vi "Initialize Module.vi"(8 "error in (no error)":errorcluster, 9 "Initialize on Error?":bool, 10 "configuration in":refnum<class "TBM module configuration.lvclass">, 11 "TBM module execution interface in":refnum<class "TBM module execution interface.lvclass">) -> (0 "error out":errorcluster, 1 "data allocations":T2, 2 "execution settings":T1, 3 "TBM module execution interface out":refnum<class "TBM module execution interface.lvclass">)   [LabVIEW 2013, in "Standard Engine Runtime.lvclass"]
uses:
  Standard Engine Runtime.lvclass
  <vilib>/NI/Tag Bus Module Framework/module configuration/TBM module configuration.lvclass
  <vilib>/NI/Tag Bus Module Framework/runtime/TBM module execution interface.lvclass
  <vilib>/NI/Tag Bus Module Framework/channel/data tables.ctl
  <vilib>/NI/Tag Bus/dictionary/data dictionary.lvclass
  <vilib>/NI/Tag Bus/dictionary table pair.ctl
  <vilib>/NI/Tag Bus/table/data table.ctl
  <vilib>/NI/Tag Bus Module Framework/runtime/execution settings.ctl
  <vilib>/NI/Tag Bus/table/data table.lvlib
  <vilib>/NI/Tag Bus/tag bus.lvlib
  <vilib>/NI/Tag Bus Module Framework/channel/TBM channel.lvclass
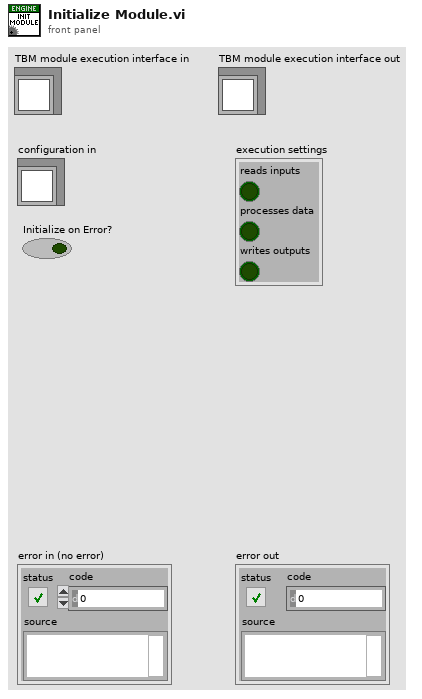
[diagram p1: front panel]
types:
  T1 = typedef "TBM module execution interface.lvclass/execution settings.ctl" = cluster{"reads inputs":bool, "processes data":bool, "writes outputs":bool}
  T2 = typedef "TBM channel.lvclass/data tables.ctl" = cluster{"input data":T3, "processing parameter":T3, "processing result":T3, "output data":T3}
  T3 = typedef "tag bus.lvlib/dictionary table pair.ctl" = cluster{"data dictionary":refnum<class "data dictionary.lvclass">, "data table":T4}
  T4 = typedef "tag bus.lvlib/data table.lvlib/data table.ctl" = cluster{"Double":dbl[], "Single":sgl[], "I64":i64[], "I32":i32[], "I16":i16[], "I8":i8[], "U64":u64[], "U32":u32[], "U16":u16[], "U8":u8[], "Boolean":bool[], "String":string[], "Array of Double":cluster{"DBL Array":dbl[]}[], "Array of Single":cluster{"SGL Array":sgl[]}[], "Array of I64":cluster{"I64 Array":i64[]}[], "Array of I32":cluster{"I32 Array":i32[]}[], "Array of I16":cluster{"I16 Array":i16[]}[], "Array of I8":cluster{"I8 Array":i8[]}[], "Array of U64":cluster{"U64 Array":u64[]}[], "Array of U32":cluster{"U32 Array":u32[]}[], "Array of U16":cluster{"U16 Array":u16[]}[], "Array of U8":cluster{"U8 Array":u8[]}[], "Array of Boolean":cluster{"Boolean Array":bool[]}[], "Array of String":cluster{"String Array":string[]}[]}
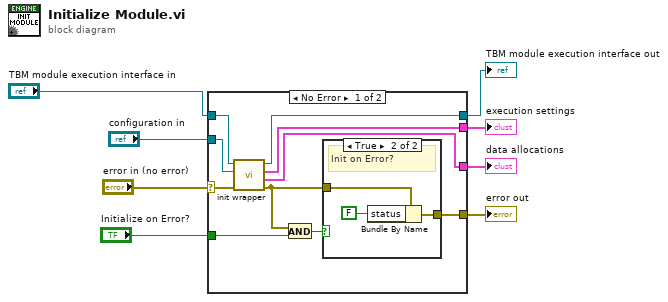
[diagram p0: block diagram]
diagram:
  n1 = case shown="No Error" "error in (no error)" {
    selector: "error in (no error)" -> [w9 w24]
    tunnel: [w18 w24] -> w8
    tunnel: "Initialize on Error?" -> [w15 _]
    tunnel: "configuration in" -> [w14 _]
    tunnel: [w13 w23] -> w5
    tunnel: [w12 _] -> w4
    tunnel: [w11 _] -> w3
    tunnel: "TBM module execution interface in" -> [w10 w23]
    frame No Error {
      n2 = call <vilib>:"init wrapper.vi"("error in (no error)"=w9, "module configuration"=w14, "module in"=w10) -> ("error out"=w17:errorcluster, "data allocations"=w12:T2, "execution settings"=w11:T1, "module out"=w13:refnum<class "TBM module execution interface.lvclass">)  [unwired: 5 in]
      n3 = And(x=w17, y=w15) -> (x .and. y?=w16:bool)
      n4 = case shown="True" w16 {
        tunnel: w17 -> [w19 w22]
        tunnel: [w19 w20] -> w18
        frame False {
        }
        frame True {
          # "Init on Error?"
          n5 = Bundle By Name(cluster=w22, "status"=FALSE) -> (w20:errorcluster)
        }
      }
    }
    frame Error {
    }
  }
  "error out" <- w8
  "TBM module execution interface out" <- w5
  "data allocations" <- w4
  "execution settings" <- w3
